vi "mod_Complex Modulator Passband.vi"(0 "x":cdb[](array[numeric]) format="%.2f", 1 "fs":dbl format="%.2f", 2 "fc":dbl format="%.2f", 3 "initial phase":dbl format="%.2f", 4 "reset?":bool) -> (5 "y":dbl[](array[numeric]) format="%.2f")   [LabVIEW 2020, in "niAMT.lvlib"]
uses:
  <vilib>/addons/Modulation/niAMT.lvlib
panel:
  # "Complex Modulator Passband"
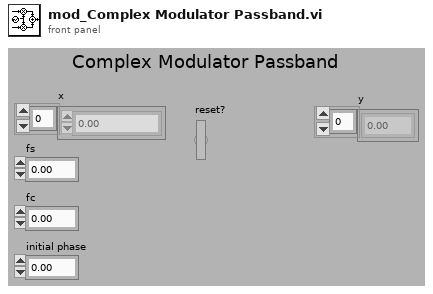
[diagram p1: front panel]
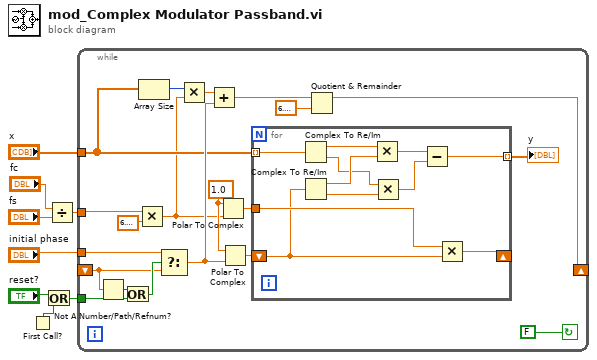
[diagram p0: block diagram]
diagram:
  n1 = First Call?() -> (First Call?: T/F=w7:bool)
  n2 = Or(x="reset?", y=w7) -> (x .or. y?=w5:bool)
  n3 = Divide(x="fc", y="fs") -> (x/y=w1:dbl)
  n4 = while {
    tunnel: w1 -> [w27]
    tunnel: "initial phase" -> [w28]
    tunnel: w5 -> [w9]
    shift-left: _ -> [w11]
    shift-right: [w14] -> _
    tunnel: "x" -> [w20]
    stop <- FALSE continue-if-true
    w22 = 1.0 ("r")
    n5 = Not A Number/Path/Refnum?(number/path/refnum=w11) -> (NaN/Path/Refnum?=w10:bool)
    n6 = Or(x=w10, y=w9) -> (x .or. y?=w12:bool)
    n7 = Multiply(x=w27, y=6.283185307179586) -> (x*y=w17:dbl)
    n8 = Array Size(array=w20) -> (size(s)=w18:i32)
    n9 = Select(t=w28, s=w12, f=w11) -> (s? t:f=w21:dbl)
    n10 = Multiply(x=w18, y=w17) -> (x*y=w19:dbl)
    n11 = Add(x=w19, y=w21) -> (x+y=w16:dbl)
    n12 = Polar To Complex(1:w17, 2:w22) -> (0:w23:cdb)
    n13 = Polar To Complex(1:w21, 2:w22) -> (0:w25:cdb)
    n14 = for {
      tunnel: w20 -> [w39] mode=indexing
      shift-right: [w30] -> _
      shift-left: w25 -> [w29]
      tunnel: [w34] -> w24 mode=indexing
      tunnel: w23 -> [w33]
      n15 = Complex To Re/Im(x + iy=w39) -> (x=w32:dbl, y=w31:dbl)
      n16 = Complex To Re/Im(x + iy=w29) -> (x=w38:dbl, y=w37:dbl)
      n17 = Multiply(x=w32, y=w38) -> (x*y=w36:dbl)
      n18 = Multiply(x=w31, y=w37) -> (x*y=w35:dbl)
      n19 = Subtract(x=w36, y=w35) -> (x-y=w34:dbl)
      n20 = Multiply(x=w33, y=w29) -> (x*y=w30:cdb)
    }
    "y" <- w24
    n21 = Quotient & Remainder(x=w16, y=6.283185307179586) -> (x-y*floor(x/y)=w14:dbl)  [unwired: 1 out]
  }
